vi "4b_bin2dec.vi"(8 "Right":bool, 9 "Left":bool, 10 "Down":bool, 11 "Up":bool) -> (2 "Out":dbl)   [LabVIEW 2012]
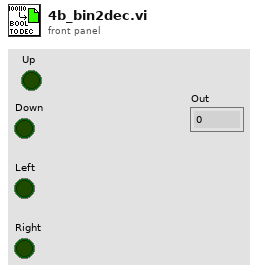
[diagram p1: front panel]
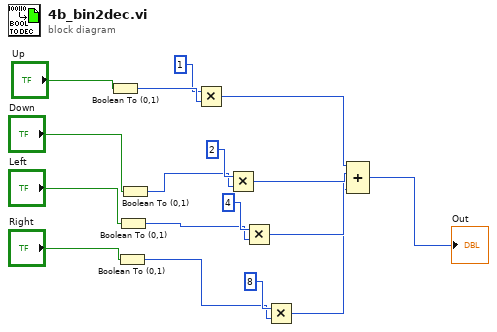
[diagram p0: block diagram]
diagram:
  n1 = Boolean To (0,1)(Boolean="Up") -> (0, 1=w13:i16)
  n2 = Boolean To (0,1)(Boolean="Right") -> (0, 1=w6:i16)
  n3 = Boolean To (0,1)(Boolean="Left") -> (0, 1=w8:i16)
  n4 = Boolean To (0,1)(Boolean="Down") -> (0, 1=w10:i16)
  n5 = Multiply(x=i16 1, y=w13) -> (x*y=w5:i16)
  n6 = Multiply(x=i16 2, y=w10) -> (x*y=w4:i16)
  n7 = Multiply(x=i16 4, y=w8) -> (x*y=w3:i16)
  n8 = Multiply(x=i16 8, y=w6) -> (x*y=w2:i16)
  n9 = Compound Arithmetic op=ADD(w5, w4, w3, w2) -> (→"Out":i16)
